vi "create INIScoreFile.vi"(8 "error in (no error)":errorcluster, 9 "Max Count (10)":i32=10, 10 "Path":path, 11 "INIScoreFile in":refnum<class "INIScoreFile.lvclass">) -> (0 "error out":errorcluster, 3 "INIScoreFile out":refnum<class "INIScoreFile.lvclass">)   [LabVIEW 2020, in "INIScoreFile.lvclass"]
uses:
  INIScoreFile.lvclass
  INIScoreFile.lvclass/INIScoreFile.ctl
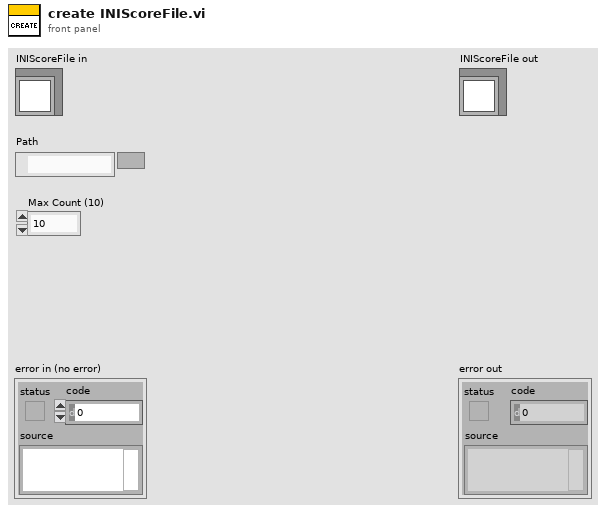
[diagram p1: front panel]
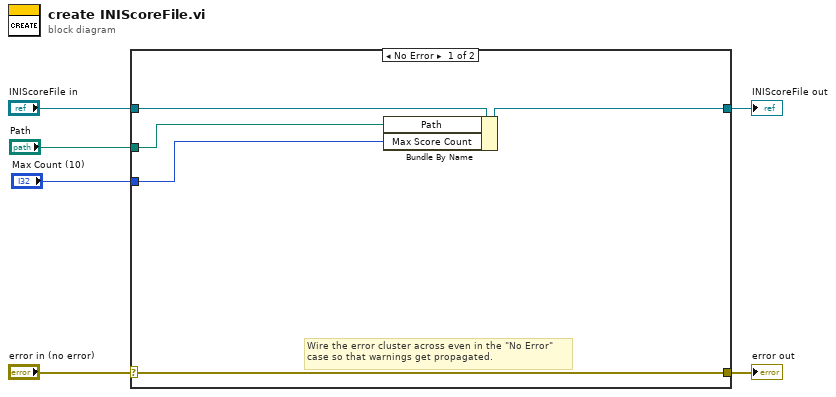
[diagram p0: block diagram]
diagram:
  n1 = case shown="No Error" "error in (no error)" {
    selector: "error in (no error)" -> [w10 w13]
    tunnel: [w10 w13] -> w5
    tunnel: [w9 w12] -> w3
    tunnel: "INIScoreFile in" -> [w11 w12]
    tunnel: "Path" -> [w8 _]
    tunnel: "Max Count (10)" -> [w7 _]
    frame No Error {
      # "Wire the error cluster across even in the \"No Error\"\ncase so that warnings get propagated."
      n2 = Bundle By Name(cluster=w11, "Path"=w8, "Max Score Count"=w7) -> (w9:refnum<class "INIScoreFile.lvclass">)
    }
    frame Error {
    }
  }
  "error out" <- w5
  "INIScoreFile out" <- w3
